vi "Update_FBFilter.vi"(7 "Axis":i32=1 min=0 max=3, 8 "error in (no error)":errorcluster, 9 "Disable?":enum16{"Disable", "Set"}(ring), 10 "Feedback Filter Settings":T1, 11 "VISA resource name":refnum<visa-resource-name>) -> (0 "error out":errorcluster, 3 "VISA resource name out":refnum<visa-resource-name>)   [LabVIEW 2011]
uses:
  <instrlib>/Newport ESP301/Newport ESP301.lvlib
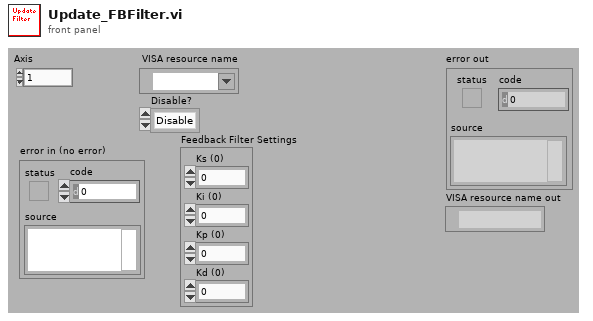
[diagram p1: front panel]
types:
  T1 = cluster{"Ks (0)":dbl, "Ki (0)":dbl, "Kp (0)":dbl, "Kd (0)":dbl}
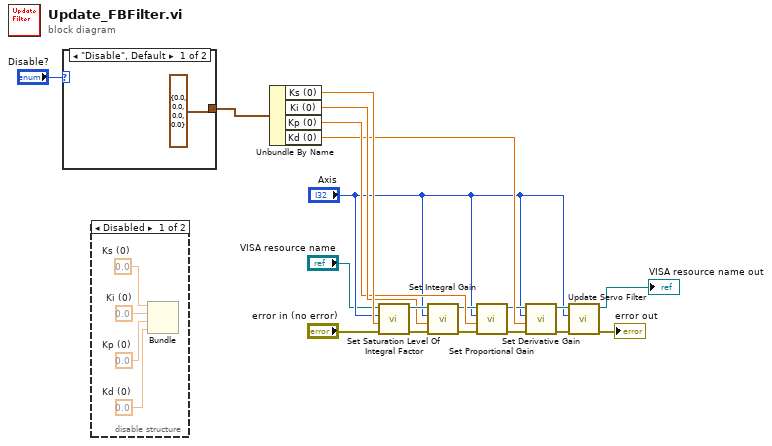
[diagram p0: block diagram]
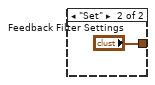
[diagram p2: hidden frame]
diagram:
  n1 = case shown="\"Disable\", Default" "Disable?" {
    tunnel: [T1 {"Ks (0)"=0.0, "Ki (0)"=0.0, "Kp (0)"=0.0, "Kd (0)"=0.0} ("output cluster") "Feedback Filter Settings"] -> w1
    frame "Disable", Default {
    }
    frame "Set" {
    }
  }
  n2 = disable-structure shown="Disabled" {
    frame Disabled {
      w22 = 0.0  # Kd (0)
      w23 = 0.0  # Kp (0)
      w24 = 0.0  # Ki (0)
      w25 = 0.0  # Ks (0)
      n3 = Bundle("Ks (0)"=w25, "Ki (0)"=w24, "Kp (0)"=w23, "Kd (0)"=w22) -> ()  [unwired: 1 in, 1 out]
    }
    frame Enabled {
    }
  }
  n4 = Unbundle By Name(w1) -> ("Ks (0)"=w17:dbl, "Ki (0)"=w16:dbl, "Kp (0)"=w15:dbl, "Kd (0)"=w14:dbl)
  n5 = call <instrlib>:"Set Saturation Level Of Integral Factor.vi"("error in (no error)"="error in (no error)", "Ks (0)"=w17, "Axis (1)"="Axis", "VISA resource name"="VISA resource name") -> ("error out"=w18:errorcluster, "VISA resource name out"=w19:refnum<visa-resource-name>)  [unwired: 2 in]
  n6 = call <instrlib>:"Set Integral Gain.vi"("error in (no error)"=w18, "Ki (0)"=w16, "Axis (1)"="Axis", "VISA resource name"=w19) -> ("error out"=w8:errorcluster, "VISA resource name out"=w13:refnum<visa-resource-name>)  [unwired: 2 in]
  n7 = call <instrlib>:"Set Proportional Gain.vi"("error in (no error)"=w8, "Kp (0)"=w15, "Axis (1)"="Axis", "VISA resource name"=w13) -> ("error out"=w9:errorcluster, "VISA resource name out"=w12:refnum<visa-resource-name>)  [unwired: 2 in]
  n8 = call <instrlib>:"Set Derivative Gain.vi"("error in (no error)"=w9, "Kd (0)"=w14, "Axis (1)"="Axis", "VISA resource name"=w12) -> ("error out"=w10:errorcluster, "VISA resource name out"=w11:refnum<visa-resource-name>)  [unwired: 2 in]
  n9 = call <instrlib>:"Update Servo Filter.vi"("error in (no error)"=w10, "Axis (0)"="Axis", "VISA resource name"=w11) -> ("error out"=→"error out":errorcluster, "VISA resource name out"=→"VISA resource name out":refnum<visa-resource-name>)  [unwired: 3 in]
